vi "uintRandom.vi"(8 "Error in (no error)":errorcluster, 10 "Base (decimal)":T1=10 items=["Binary"=2, "Octal"=8, "Decimal"=10, "Hexadecimal"=16, "Hexatrigesimal"=36, "ASCII"=64], 11 "Number of decimals":i32=100) -> (0 "Error out":errorcluster, 3 "Uint out":refnum<class "UintClass.lvclass">)   [LabVIEW 2011, in "UintClass.lvclass"]
uses:
  UintClass.lvclass
  enumBase.ctl
  <userlib>/_OpenG.lib/numeric/numeric.llb/Random Number Within Range - I32__ogtk.vi
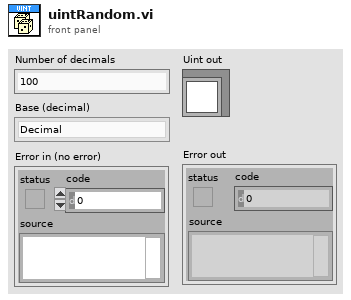
[diagram p1: front panel]
types:
  T1 = typedef "UintClass.lvclass/enumBase.ctl" = u16
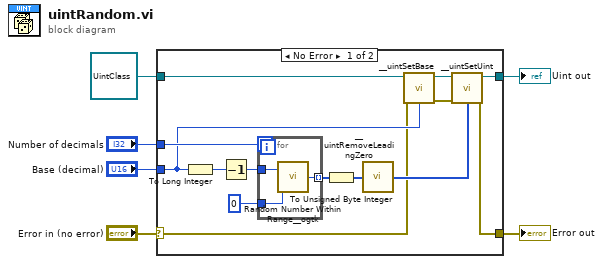
[diagram p0: block diagram]
diagram:
  n1 = case shown="No Error" "Error in (no error)" {
    selector: "Error in (no error)" -> [w7 w25]
    tunnel: refnum<class "UintClass.lvclass"> refnum ("UintClass.lvclass") -> [w8 w24]
    tunnel: "Number of decimals" -> [w20 _]
    tunnel: "Base (decimal)" -> [w9 _]
    tunnel: [w12 w25] -> w2
    tunnel: [w13 w24] -> w1
    frame No Error {
      n2 = To Long Integer(number=w9) -> (32bit integer=w19:i32)
      n3 = Decrement(x=w19) -> (x-1=w16:i32)
      n4 = for {
        N: w20 -> [_]
        tunnel: w16 -> [w23]
        tunnel: 0 ("Low") -> [w22]
        tunnel: [w21] -> w17 mode=indexing
        n5 = call-poly <userlib>:"Random Number Within Range__ogtk.vi"("High"=w23, "Low"=w22) -> ("Random Number"=w21:i32)  [unwired: 3 in]
      }
      n6 = To Unsigned Byte Integer(number=w17) -> (unsigned 8bit integer=w15:u8[])
      n7 = call "__uintRemoveLeadingZero.vi"("Uint in"=w15) -> ("Uint out"=w10:u8[])
      n8 = call "__uintSetBase.vi"("Error in (no error)"=w7, "Base (decimal)"=w9, "Uint in"=w8) -> ("Error out"=w11:errorcluster, "Uint out"=w14:refnum<class "UintClass.lvclass">)  [unwired: 7 in]
      n9 = call "__uintSetUint.vi"("Error in (no error)"=w11, 10:"Uint in"=w10, 11:"Uint in"=w14) -> ("Error out"=w12:errorcluster, "Uint out"=w13:refnum<class "UintClass.lvclass">)  [unwired: 7 in]
    }
    frame Error {
    }
  }
  "Error out" <- w2
  "Uint out" <- w1
